vi "Result_not_used.vi"(8 "error in (no error)":errorcluster, 11 "IV_data in":refnum<class "IV_data.lvclass">) -> (0 "error out":errorcluster, 3 "IV_data out":refnum<class "IV_data.lvclass">)   [LabVIEW 2014, in "IV_data.lvclass"]
uses:
  IV_data.lvclass
  <vilib>/Utility/file.llb/Write Delimited Spreadsheet (DBL).vi
panel:
  in  "path":path
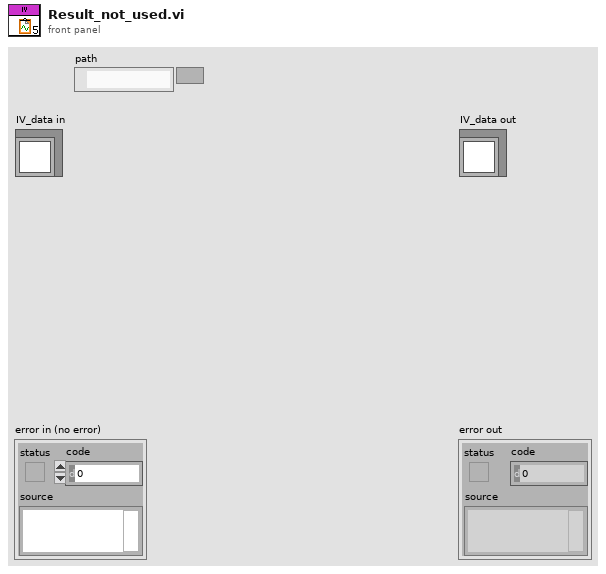
[diagram p1: front panel]
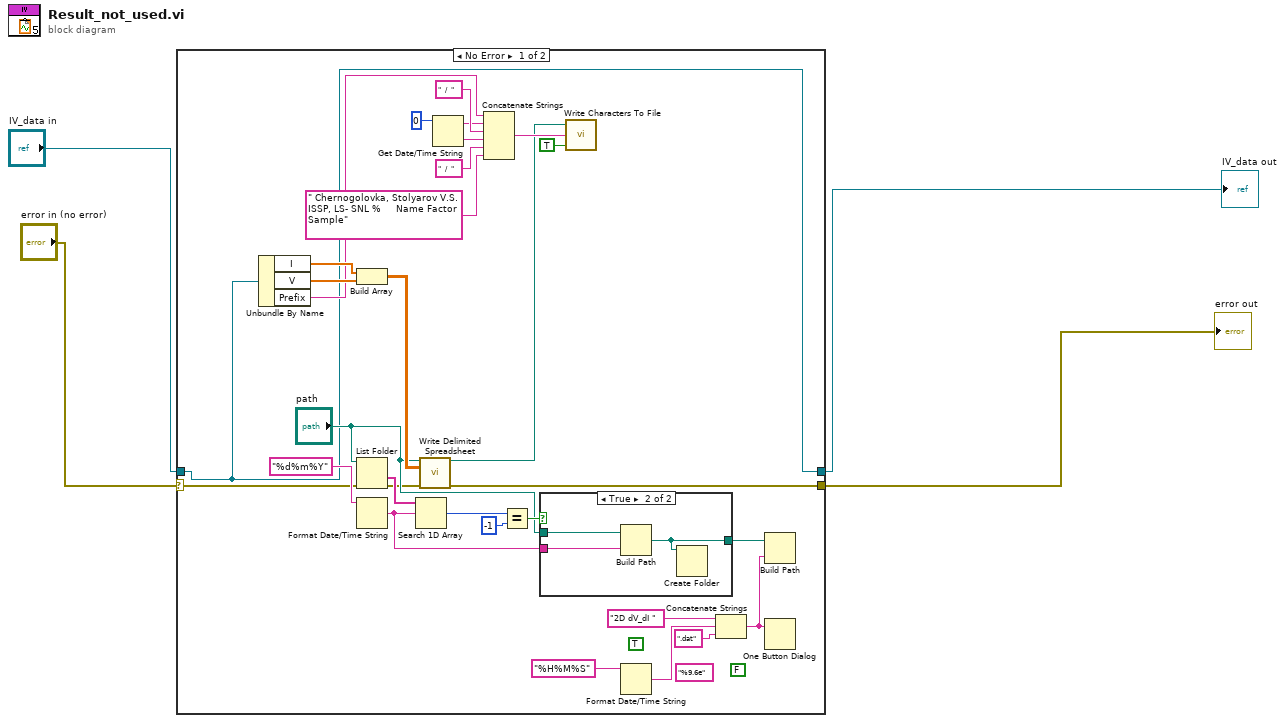
[diagram p0: block diagram]
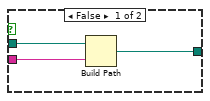
[diagram p2: hidden frame]
diagram:
  n1 = case shown="No Error" "error in (no error)" {
    selector: "error in (no error)" -> [w6 w42]
    tunnel: "IV_data in" -> [w5 w41]
    tunnel: [w8 w42] -> w3
    tunnel: [w5 w41] -> w1
    frame No Error {
      (unwired) TRUE ("transpose? (no:F)")
      (unwired) FALSE ("append to file? (new file:F)")
      (unwired) "%9.6e" ("format (%.3f)")
      n2 = Unbundle By Name(w5) -> ("I"=w14:dbl[], "V"=w13:dbl[], "Prefix"=w12:string)
      n3 = Build Array(w14, w13) -> (w11:dbl[][])
      n4 = List Folder(path="path", error in=w6) -> (folder names=w31:string[], error out=w7:errorcluster)  [unwired: 2 in, 2 out]
      n5 = Format Date/Time String(time format string (%c)="%d%m%Y") -> (date/time string=w15:string)  [unwired: 2 in]
      n6 = Search 1D Array(1D array=w31, element=w15) -> (index of element=w32:i32)  [unwired: 1 in]
      n7 = call-poly <vilib>:"Write Delimited Spreadsheet.vi"("file path (dialog if empty)"="path", "2D data"=w11, "error in (no error)"=w7) -> ("new file path (Not A Path if cancelled)"=w9:path, "error out"=w8:errorcluster)  [unwired: 11 in]
      n8 = Get Date/Time String(date format (0)=0) -> (date string=w26:string, time string=w27:string)  [unwired: 2 in]
      n9 = Concatenate Strings(w12, w26, "  /  " ("date string"), w27, "  /  " ("date string"), " Chernogolovka, Stolyarov V.S. ISSP, LS- SNL %     Name Factor Sample" ("date string")) -> (w25:string)
      n10 = Equal?(x=w32, y=-1) -> (x = y?=w34:bool)
      n11 = case shown="True" w34 {
        tunnel: w15 -> [w37 w40]
        tunnel: [w36 w39] -> w22
        tunnel: "path" -> [w35 w38]
        frame False {
          n12 = Build Path(base path=w35, name or relative path=w37) -> (appended path=w36:path)
        }
        frame True {
          n13 = Build Path(base path=w38, name or relative path=w40) -> (appended path=w39:path)
          n14 = Create Folder(path (use dialog)=w39) -> ()  [unwired: 2 in, 3 out]
        }
      }
      n15 = call <vilib>:"Write Characters To File.vi"("append to file? (new file:F)"=TRUE, "character string"=w25, "file path (dialog if empty)"=w9) -> ()  [unwired: 2 in, 1 out]
      n16 = Format Date/Time String(time format string (%c)="%H%M%S") -> (date/time string=w18:string)  [unwired: 2 in]
      n17 = Concatenate Strings("2D dV_dI " ("string"), w18, ".dat" ("substring")) -> (w21:string)
      n18 = Build Path(base path=w22, name or relative path=w21) -> ()  [unwired: 1 out]
      n19 = One Button Dialog(message=w21) -> ()  [unwired: 1 in, 1 out]
    }
    frame Error {
    }
  }
  "error out" <- w3
  "IV_data out" <- w1
